vi "Transition.vi"(8 "error in (no error)":errorcluster, 9 "Target State":refnum<class "State.lvclass">, 10 "Source State":refnum<class "State.lvclass">, 11 "Internal in":refnum<class "Internal.lvclass">) -> (0 "error out":errorcluster, 2 "State out":refnum<class "State.lvclass">, 3 "Internal out":refnum<class "Internal.lvclass">)   [LabVIEW 2024, in "Transition.lvlib" / "Internal.lvclass"]
uses:
  Internal.lvclass
  Internal.lvclass/Internal.ctl
  State/State/State.lvclass
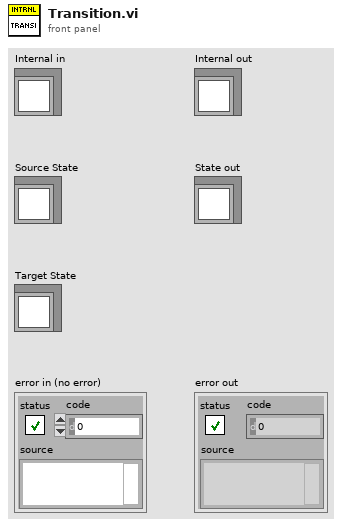
[diagram p1: front panel]
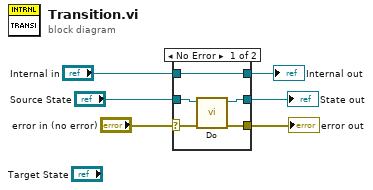
[diagram p0: block diagram]
diagram:
  n1 = case shown="No Error" "error in (no error)" {
    selector: "error in (no error)" -> [w8 w13]
    tunnel: "Source State" -> [w11 w14]
    tunnel: [w10 w14] -> w5
    tunnel: [w9 w13] -> w4
    tunnel: [w7 w12] -> w2
    tunnel: "Internal in" -> [w7 w12]
    frame No Error {
      n2 = call-dynamic "Do.vi"("error in (no error)"=w8, "State in"=w11) -> ("error out"=w9:errorcluster, "State out"=w10:refnum<class "State.lvclass">)  [unwired: 8 in]
    }
    frame Error {
    }
  }
  "error out" <- w4
  "Internal out" <- w2
  "State out" <- w5
